vi "Initialize card.vi"(8 "error in (no error)":errorcluster, 9 "Trigger Timeout (10000000)":dbl=1000.0 format="%#_13g", 10 "Control cluster 2":T1={"Number of points"=816000.0, "Input Range"=10000, "Trigger Level"=29, "Trigger source"=TRUE} {"Trigger Level" min=-60 max=60 step=1 scale=-60.0..60.0; "Input Range" items=["+/- 5 V"=10000, "+/- 2 V"=4000, "+/- 1 V"=2000, "+/- 500 mV"=1000, "+/- 200 mV"=400, "+/- 100 mV"=200]; "Number of points" min=160.0 step=160.0}, 11 "Gage digitizer actor in":refnum<class "Gage digitizer actor.lvclass">) -> (0 "error out":errorcluster, 3 "Gage digitizer actor out":refnum<class "Gage digitizer actor.lvclass">)   [LabVIEW 2015, in "Gage digitizer actor.lvclass"]
uses:
  Gage digitizer actor.lvclass
  Gage digitizer actor.lvclass/Gage digitizer actor.ctl
  Read_Pulse/Control_interface.lvclass
  Read_Pulse/Control_card.lvclass
panel:
  # "Basic Card Controlls"
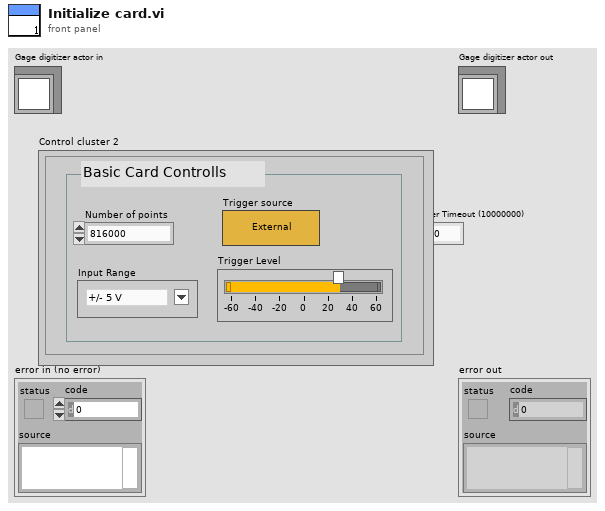
[diagram p1: front panel]
types:
  T1 = cluster{"Number of points":dbl, "Input Range":u32, "Trigger Level":i32, "Trigger source":bool}
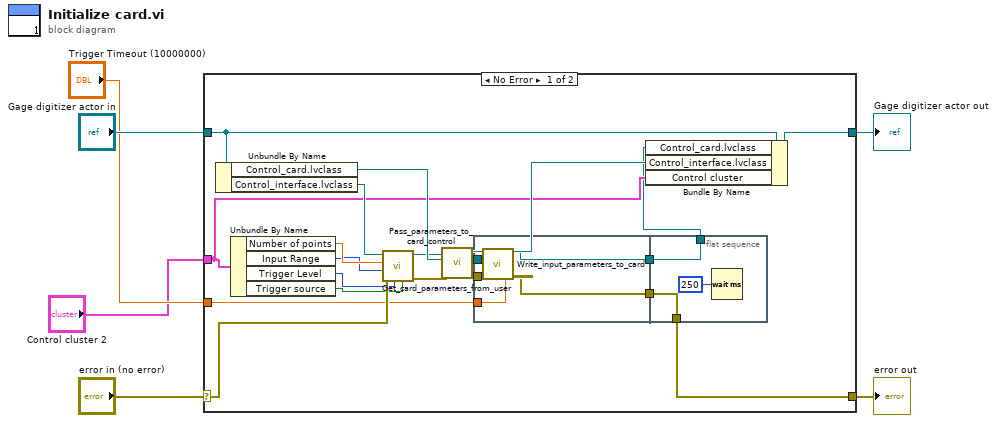
[diagram p0: block diagram]
diagram:
  n1 = case shown="No Error" "error in (no error)" {
    selector: "error in (no error)" -> [w21 w36]
    tunnel: [w7 w36] -> w5
    tunnel: [w14 w35] -> w3
    tunnel: "Gage digitizer actor in" -> [w26 w35]
    tunnel: "Control cluster 2" -> [w12 _]
    tunnel: "Trigger Timeout (10000000)" -> [w11 _]
    frame No Error {
      n2 = Unbundle By Name(w26) -> ("Control_card.lvclass"=w25:refnum<class "Control_card.lvclass">, "Control_interface.lvclass"=w24:refnum<class "Control_interface.lvclass">)
      n3 = Unbundle By Name(w12) -> ("Number of points"=w18:dbl, "Input Range"=w17:u32, "Trigger Level"=w16:i32, "Trigger source"=w15:bool)
      n4 = call-dynamic "Get_card_parameters_from_user.vi"("External Trigger?"=w15, "Trigger Level"=w16, "error in (no error)"=w21, "Range"=w17, "Number of points"=w18, "Control_interface in"=w24) -> ("error out"=w20:errorcluster, "Control_interface out"=w23:refnum<class "Control_interface.lvclass">)  [unwired: 4 in]
      n5 = call "Pass_parameters_to_card_control.vi"("error in (no error)"=w20, "Control_card.lvclass"=w25, "Control_interface in"=w23) -> ("error out"=w19:errorcluster, "Initialize_card out"=w22:refnum<class "Control_card.lvclass">, "Control_interface out"=w13:refnum<class "Control_interface.lvclass">)  [unwired: 6 in]
      n6 = flat-sequence {
        tunnel: w22 -> [w31]
        tunnel: w19 -> [w30]
        tunnel: w11 -> [w29]
        tunnel: [w28] -> w10
        tunnel: [w27] -> w8
        tunnel: w10 -> [w34]
        tunnel: [w34] -> w9
        tunnel: w8 -> [w33]
        tunnel: [w33] -> w7
        frame #0 {
          n7 = call "Write_input_parameters_to_card.vi"("error in (no error)"=w30, "Trigger Timeout (10000000)"=w29, "Control_card in"=w31) -> ("error out"=w27:errorcluster, "Control_card out"=w28:refnum<class "Control_card.lvclass">)  [unwired: 7 in]
        }
        frame #1 {
          n8 = Wait (ms)(milliseconds to wait=u32 250) -> ()  [unwired: 1 out]
        }
      }
      n9 = Bundle By Name(cluster=w26, "Control_card.lvclass"=w9, "Control_interface.lvclass"=w13, "Control cluster"=w12) -> (w14:refnum<class "Gage digitizer actor.lvclass">)
    }
    frame Error {
    }
  }
  "error out" <- w5
  "Gage digitizer actor out" <- w3
